vi "Periodic Tasks.vi"(8 "error in":errorcluster) -> ()   [LabVIEW 2018]
doc: "This VI runs in parallel to other robot code. It can contain as many user-defined periodic loops as you need. These can carry out PID or other sorts of timed response."
uses:
  Robot Global Data.vi
panel:
  out "Cargo Stop Current":dbl=10.0 format="%#_13g"
  out "Stop the grabber":bool
  out "Solenoid Voltage":dbl
  out "Input Voltage":dbl
  out "Compressor current (A)":dbl
  out "all currents (A)":dbl[](array[numeric]) caption="0\n1\n2\n3\n4\n5\n6\n7\n8\n9\n10\n11\n12\n13\n14\n15"
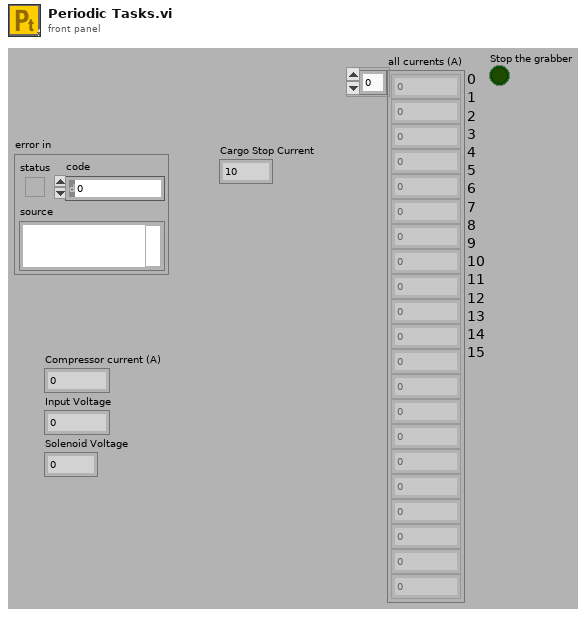
[diagram p1: front panel]
types:
  T1 = typedef "WPI_JoystickDevRef.ctl" = cluster{"Device":T2}
  T2 = typedef "WPI_JoystickDeviceEnum.ctl" = enum16{"USB 0", "USB 1", "USB 2", "USB 3", "USB 4", "USB 5"}
  T3 = cluster{"JoystickDevRef":T1, "JoystickDevRef":T1}
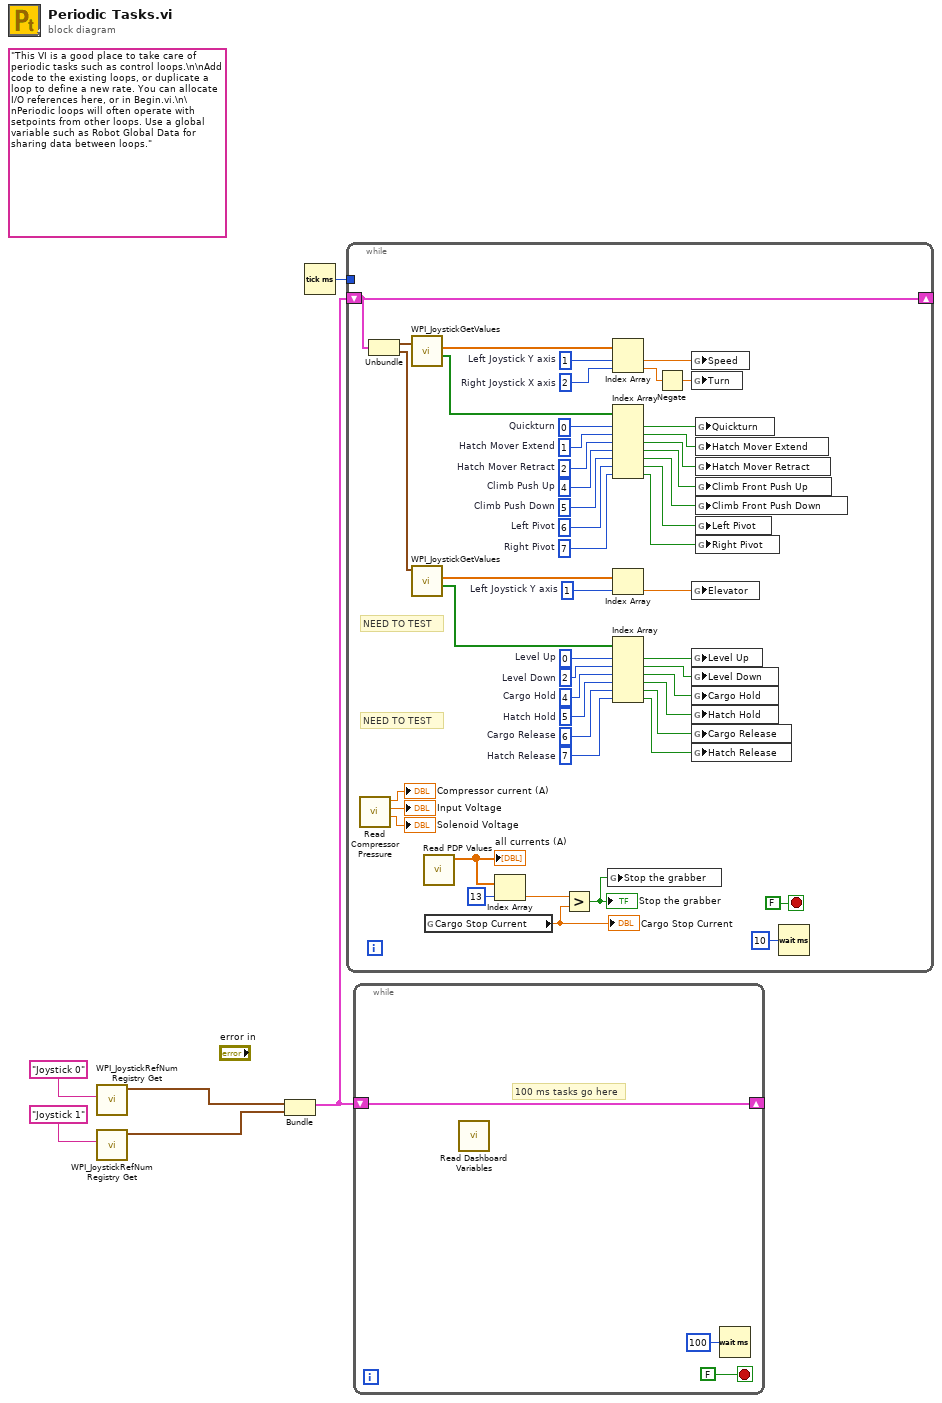
[diagram p0: block diagram]
diagram:
  (unwired) "This VI is a good place to take care of periodic tasks such as control loops.\n\nAdd code to the existing loops, or duplicate a loop to define a new rate. You can allocate I/O references here, or in Begin.vi.\n\nPeriodic loops will often operate with setpoints from other loops. Use a global variable such as Robot Global Data for sharing data between loops."
  n1 = call <vilib>:"WPI_JoystickRefNum Registry Get.vi"("refnum name"="Joystick 0") -> ("JoystickDevRef"=w3:T1)  [unwired: 1 in, 9 out]
  n2 = call <vilib>:"WPI_JoystickRefNum Registry Get.vi"("refnum name"="Joystick 1") -> ("JoystickDevRef"=w1:T1)  [unwired: 1 in, 9 out]
  n3 = Bundle("JoystickDevRef"=w3, "JoystickDevRef"=w1) -> (w2:T3)  [unwired: 1 in]
  n4 = Tick Count (ms)() -> (millisecond timer value=w5:u32)
  n5 = while {
    shift-right: [w51] -> _
    shift-left: w2 -> [w51]
    tunnel: w5 -> [_]
    stop <- FALSE stop-if-true
    w10 = 7  # Right Pivot
    w9 = 6  # Left Pivot
    w16 = 5  # Climb Push Down
    w17 = 4  # Climb Push Up
    w24 = 7  # Hatch Release
    w25 = 6  # Cargo Release
    w26 = 5  # Hatch Hold
    w27 = 4  # Cargo Hold
    w28 = 2  # Level Down
    w29 = 0  # Level Up
    w32 = 1  # Left Joystick Y axis
    w33 = 2  # Hatch Mover Retract
    w34 = 1  # Hatch Mover Extend
    w35 = 0  # Quickturn
    w45 = 2  # Right Joystick X axis
    w46 = 1  # Left Joystick Y axis
    # "NEED TO TEST"
    # "NEED TO TEST"
    n6 = call "Read Compressor Pressure.vi"() -> ("Solenoid Voltage"=→"Solenoid Voltage":dbl, "Input Voltage"=→"Input Voltage":dbl, "Compressor current (A)"=→"Compressor current (A)":dbl)  [unwired: 9 in]
    n7 = Unbundle(w51) -> ("JoystickDevRef"=w50:T1, "JoystickDevRef"=w47:T1)
    n8 = call <vilib>:"WPI_JoystickGetValues.vi"("JoystickDevRef"=w50) -> ("Buttons"=w52:bool[], "Axes"=w54:dbl[])  [unwired: 6 in, 3 out]
    n9 = call <vilib>:"WPI_JoystickGetValues.vi"("JoystickDevRef"=w47) -> ("Buttons"=w49:bool[], "Axes"=w48:dbl[])  [unwired: 6 in, 3 out]
    n10 = call "Read PDP Values.vi"() -> ("all currents (A)"=w37:dbl[])  [unwired: 11 in]
    "all currents (A)" <- w37
    n11 = global read "Robot Global Data.vi" "Cargo Stop Current"() -> (w30:dbl)
    "Cargo Stop Current" <- w30
    n12 = Index Array(array=w37, index=13) -> (element=w39:dbl)
    n13 = Greater?(x=w39, y=w30) -> (0:w36:bool)
    "Stop the grabber" <- w36
    n14 = global write "Robot Global Data.vi" "Stop the grabber"(w36) -> ()
    n15 = Index Array(array=w54, index #1=w46, index #2=w45) -> (element #1=w44:dbl, element #2=w43:dbl)
    n16 = Index Array(array=w52, index #1=w35, index #2=w34, index #3=w33, index #4=w17, index #5=w16, index #6=w9, index #7=w10) -> (element #1=w15:bool, element #2=w14:bool, element #3=w13:bool, element #4=w12:bool, element #5=w11:bool, element #6=w7:bool, element #7=w8:bool)
    n17 = Index Array(array=w48, index=w32) -> (element=w31:dbl)
    n18 = Index Array(array=w49, index #1=w29, index #2=w28, index #3=w27, index #4=w26, index #5=w25, index #6=w24) -> (element #1=w23:bool, element #2=w22:bool, element #3=w21:bool, element #4=w20:bool, element #5=w19:bool, element #6=w18:bool)
    n19 = Negate(x=w43) -> (-x=w53:dbl)
    n20 = global write "Robot Global Data.vi" "Speed"(w44) -> ()
    n21 = global write "Robot Global Data.vi" "Turn"(w53) -> ()
    n22 = global write "Robot Global Data.vi" "Elevator"(w31) -> ()
    n23 = global write "Robot Global Data.vi" "Level Up"(w23) -> ()
    n24 = global write "Robot Global Data.vi" "Level Down"(w22) -> ()
    n25 = global write "Robot Global Data.vi" "Cargo Hold"(w21) -> ()
    n26 = global write "Robot Global Data.vi" "Hatch Hold"(w20) -> ()
    n27 = global write "Robot Global Data.vi" "Cargo Release"(w19) -> ()
    n28 = global write "Robot Global Data.vi" "Hatch Release"(w18) -> ()
    n29 = global write "Robot Global Data.vi" "Quickturn"(w15) -> ()
    n30 = global write "Robot Global Data.vi" "Hatch Mover Extend"(w14) -> ()
    n31 = global write "Robot Global Data.vi" "Hatch Mover Retract"(w13) -> ()
    n32 = global write "Robot Global Data.vi" "Climb Front Push Up"(w12) -> ()
    n33 = global write "Robot Global Data.vi" "Climb Front Push Down"(w11) -> ()
    n34 = global write "Robot Global Data.vi" "Left Pivot"(w7) -> ()
    n35 = global write "Robot Global Data.vi" "Right Pivot"(w8) -> ()
    n36 = Wait (ms)(milliseconds to wait=u32 10) -> ()  [unwired: 1 out]
  }
  n37 = while {
    shift-right: [w57] -> _
    shift-left: w2 -> [w57]
    stop <- FALSE stop-if-true
    # "100 ms tasks go here"
    n38 = call "Read Dashboard Variables.vi"() -> ()  [unwired: 12 in]
    n39 = Wait (ms)(milliseconds to wait=u32 100) -> ()  [unwired: 1 out]
  }
